vi "Move to point.vi"(7 "Speed":dbl, 11 "array":string) -> ()   [LabVIEW 2011]
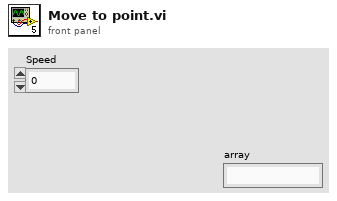
[diagram p1: front panel]
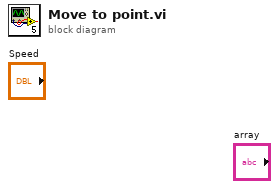
[diagram p0: block diagram]
diagram:
